vi "error handler.vi"(7 "function (unspecified)":T1(ring), 8 "error in":errorcluster, 10 "errno number":i32, 11 "errno":T2(ring)) -> (0 "error out":errorcluster)   [LabVIEW 2018, in "PCANBasic.lvlib" / "epoll.lvclass"]
uses:
  epoll.lvclass
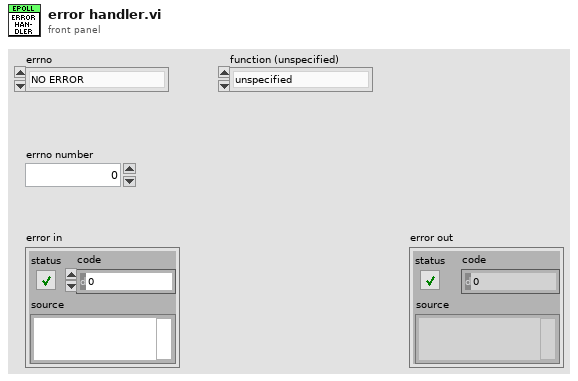
[diagram p1: front panel]
types:
  T1 = enum16{"unspecified", "close", "epoll_create", "epoll_ctl", "epoll_wait"}
  T2 = enum16{"NO ERROR", "EPERM", "ENOENT", "ESRCH", "EINTR", "EIO", "ENXIO", "E2BIG", "ENOEXEC", "EBADF", "ECHILD", "EAGAIN", "ENOMEM", "EACCES", "EFAULT", "ENOTBLK", "EBUSY", "EEXIST", "EXDEV", "ENODEV", "ENOTDIR", "EISDIR", "EINVAL", "ENFILE", "EMFILE", "ENOTTY", "ETXTBSY", "EFBIG", "ENOSPC", "ESPIPE", "EROFS", "EMLINK", "EPIPE", "EDOM", "ERANGE", "EDADLK", "ENAMETOOLONG", "ENOLCK", "ENOSYS", "ENOTEMPTY", "ELOOP", "EWOULDBLOCK", "ENOMSG", "EIDRM", "ECHRNG", "EL2NSYNC", "EL3HLT", "EL3RST", "ELNRNG", "EUNATCH", "ENOCSI", "EL2HLT", "EBADE", "EBADR", "EXFULL", "ENOANO", "EBADRQC", "EBADSLT", "EDEADLOCK", "EBFONT", "ENOSTR", "ENODATA", "ETIME", "ENOSR", "ENONET", "ENOPKG", "EREMOTE", "ENOLINK", "EADV", "ESRMNT", "ECOMM", "EPROTO", "EMULTIHOP", "EDOTDOT", "EBADMSG", "EOVERFLOW", "ENOTUNIQ", "EBADFD", "EREMCHG", "ELIBACC", "ELIBBAD", "ELIBSCN", "ELIBMAX", "ELIBEXEC", "ELISEQ", "ERESTART", "ESTRPIPE", "EUSERS", "ENOTSOCK", "EDESTADDRREQ", "EMSGSIZE", "EPROTOTYPE", "ENOPROTOOPT", "EPROTONOSUPPORT", "ESOCKTNOSUPPORT", "EOPNOTSUPP", "EPFNOSUPPORT", "EAFNOSUPPORT", "EADDRINUSE", "EADDRNOTAVAIL", "ENETDOWN", "ENETUNREACH", "ENETRESET", "ECONNABORTED", "ECONNRESET", "ENOBUFS", "EISCONN", "ENOTCONN", "ESHUTDOWN", "ETOOMANYREFS", "ETIMEDOUT", "ECONNREFUSED", "EHOSTDOWN", "EHOSTUNREACH", "EALREADY", "EINPROGRESS", "ESTALE", "EUCLEAN", "ENOTNAM", "ENAVAIL", "EISNAM", "EREMOTEIO", "EDQUOT", "ENOMEDIUM", "EMEDIUMTYPE", "ECANCELED", "ENOKEY", "EKEYEXPIRED", "EKEYREVOKED", "EKEYREJECTED", "EOWNERDEAD", "ENOTRECOVERABLE", "ERFKILL", "EHWPOISON", "UNDEFINED"}
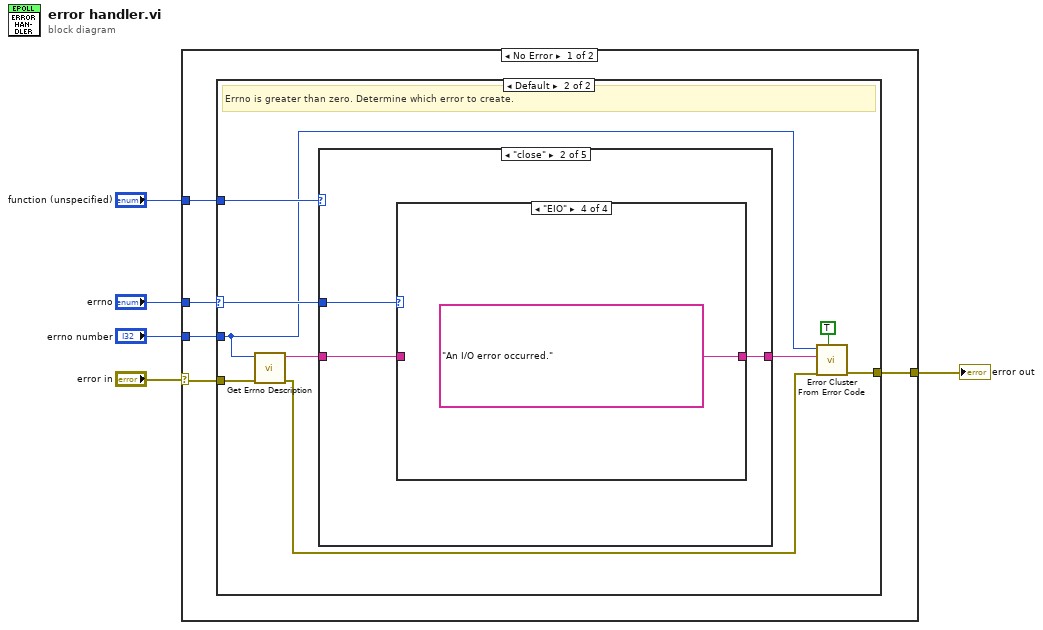
[diagram p0: block diagram]
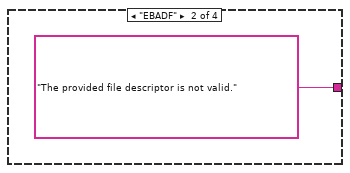
[diagram p5: hidden frame]
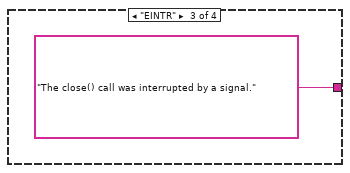
[diagram p6: hidden frame]
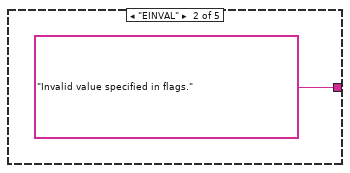
[diagram p8: hidden frame]
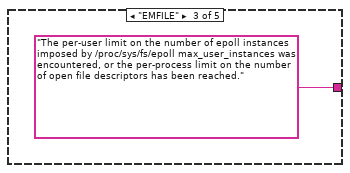
[diagram p9: hidden frame]
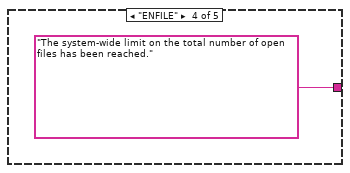
[diagram p10: hidden frame]
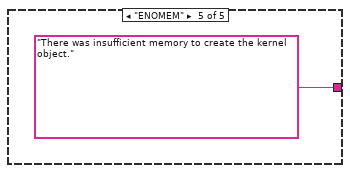
[diagram p11: hidden frame]
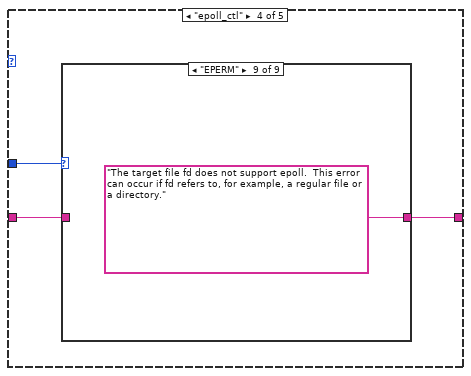
[diagram p12: hidden frame]
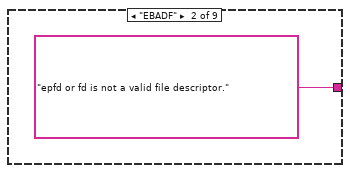
[diagram p14: hidden frame]
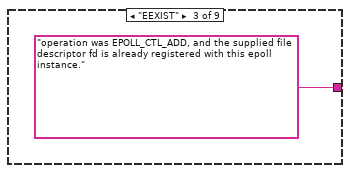
[diagram p15: hidden frame]
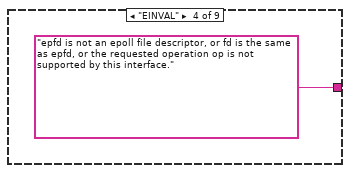
[diagram p16: hidden frame]
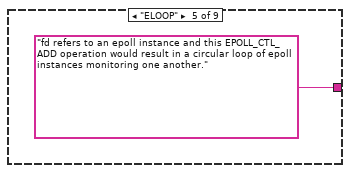
[diagram p17: hidden frame]
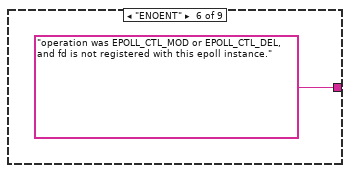
[diagram p18: hidden frame]
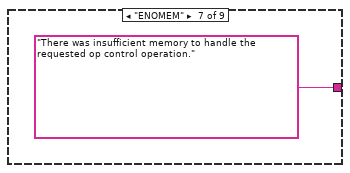
[diagram p19: hidden frame]
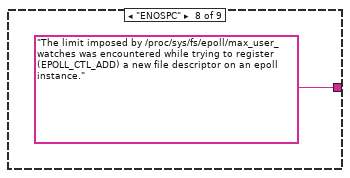
[diagram p20: hidden frame]
diagram:
  n1 = case shown="No Error" "error in" {
    selector: "error in" -> [w6 w56]
    tunnel: [w10 w56] -> w4
    tunnel: "errno" -> [w8 _]
    tunnel: "function (unspecified)" -> [w9 _]
    tunnel: "errno number" -> [w7 _]
    frame No Error {
      n2 = case shown="Default" w8 {
        selector: w8 -> [_ w15]
        tunnel: [_ w19] -> w10
        tunnel: w9 -> [_ w17]
        tunnel: w7 -> [_ w11]
        tunnel: w6 -> [_ w14]
        frame "NO ERROR" {
          # "Errno is zero. No error occurred."
        }
        frame Default {
          # "Errno is greater than zero. Determine which error to create."
          n3 = call "Get Errno Description.vi"("error in"=w14, "errnum"=w11) -> ("error out"=w13:errorcluster, "Description"=w12:string)  [unwired: 8 in]
          n4 = case shown="\"close\"" w17 {
            tunnel: w15 -> [_ w21 w30 w38 w50]
            tunnel: [w20 w23 w29 w37 w49] -> w16
            tunnel: w12 -> [w20 w22 w28 w36 w48]
            frame "unspecified", Default {
              # "No specific function was specified, so use generic error description."
            }
            frame "close" {
              n5 = case shown="\"EIO\"" w21 {
                tunnel: [w24 "The provided file descriptor is not valid." "The close() call was interrupted by a signal." "An I/O error occurred."] -> w23
                tunnel: w22 -> [w24 _ _ _]
                frame "NO ERROR", Default {
                }
                frame "EBADF" {
                }
                frame "EINTR" {
                }
                frame "EIO" {
                }
              }
            }
            frame "epoll_create" {
              n6 = case shown="\"NO ERROR\", Default" w30 {
                tunnel: [w31 "Invalid value specified in flags." "The per-user limit on the number of epoll instances imposed by /proc/sys/fs/epoll max_user_instances was encountered, or the per-process limit on the number of open file descriptors has been reached." "The system-wide limit on the total number of open files has been reached." "There was insufficient memory to create the kernel object."] -> w29
                tunnel: w28 -> [w31 _ _ _ _]
                frame "NO ERROR", Default {
                }
                frame "EINVAL" {
                }
                frame "EMFILE" {
                }
                frame "ENFILE" {
                }
                frame "ENOMEM" {
                }
              }
            }
            frame "epoll_ctl" {
              n7 = case shown="\"EPERM\"" w38 {
                tunnel: [w39 "epfd or fd is not a valid file descriptor." "operation was EPOLL_CTL_ADD, and the supplied file descriptor fd is already registered with this epoll instance." "epfd is not an epoll file descriptor, or fd is the same as epfd, or the requested operation op is not supported by this interface." "fd refers to an epoll instance and this EPOLL_CTL_ADD operation would result in a circular loop of epoll instances monitoring one another." "operation was EPOLL_CTL_MOD or EPOLL_CTL_DEL, and fd is not registered with this epoll instance." "There was insufficient memory to handle the requested op control operation." "The limit imposed by /proc/sys/fs/epoll/max_user_watches was encountered while trying to register (EPOLL_CTL_ADD) a new file descriptor on an epoll instance." "The target file fd does not support epoll.  This error can occur if fd refers to, for example, a regular file or a directory."] -> w37
                tunnel: w36 -> [w39 _ _ _ _ _ _ _ _]
                frame "NO ERROR", Default {
                }
                frame "EBADF" {
                }
                frame "EEXIST" {
                }
                frame "EINVAL" {
                }
                frame "ELOOP" {
                }
                frame "ENOENT" {
                }
                frame "ENOMEM" {
                }
                frame "ENOSPC" {
                }
                frame "EPERM" {
                }
              }
            }
            frame "epoll_wait" {
              n8 = case shown="\"EINVAL\"" w50 {
                tunnel: [w51 "epfd is not a valid file descriptor." "The memory area pointed to by events is not write permissions." "The call was interrupted by a signal handler before either (1) any of the requested events occurred or (2) the timeout expired." "epfd is not an epoll file descriptor, or maxevents is less than or equal to zero."] -> w49
                tunnel: w48 -> [w51 _ _ _ _]
                frame "NO ERROR", Default {
                }
                frame "EBADF" {
                }
                frame "EFAULT" {
                }
                frame "EINTR" {
                }
                frame "EINVAL" {
                }
              }
            }
          }
          n9 = call <vilib>:"Error Cluster From Error Code.vi"("show call chain? (False)"=TRUE, "error in (no error)"=w13, "error message (\"\")"=w16, "error code (0)"=w11) -> ("error out"=w19:errorcluster)  [unwired: 5 in]
        }
      }
    }
    frame Error {
      # "Error already exists. Pass through."
    }
  }
  "error out" <- w4
